vi "Client2.vi"() -> ()   [LabVIEW 2019]
panel:
  out "Connected":bool
  out "error out":errorcluster
  in  "UserName :":string
  in  "JOIN":bool
  in  "Message":string
  in  "SEND Button":bool
  in  "?":bool
  out "Chat Screen":string
  # "Welcome to Chat Application\nPlease type a username and click \"JOIN\" to join the chat room.\nYou can send your message  in \"Message Box\" with \"SEND MESSAGE\" button.\nAnd you can leave the chat room with \"QUIT\" button.\nIf you want to Join the chat room again, you should stop and run program again."
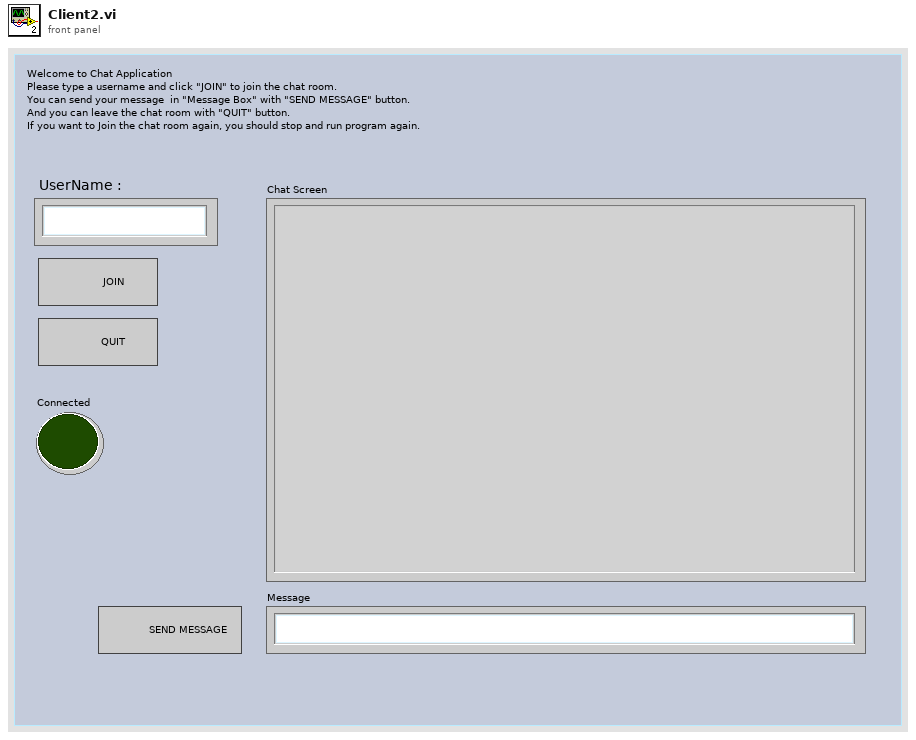
[diagram p1: front panel]
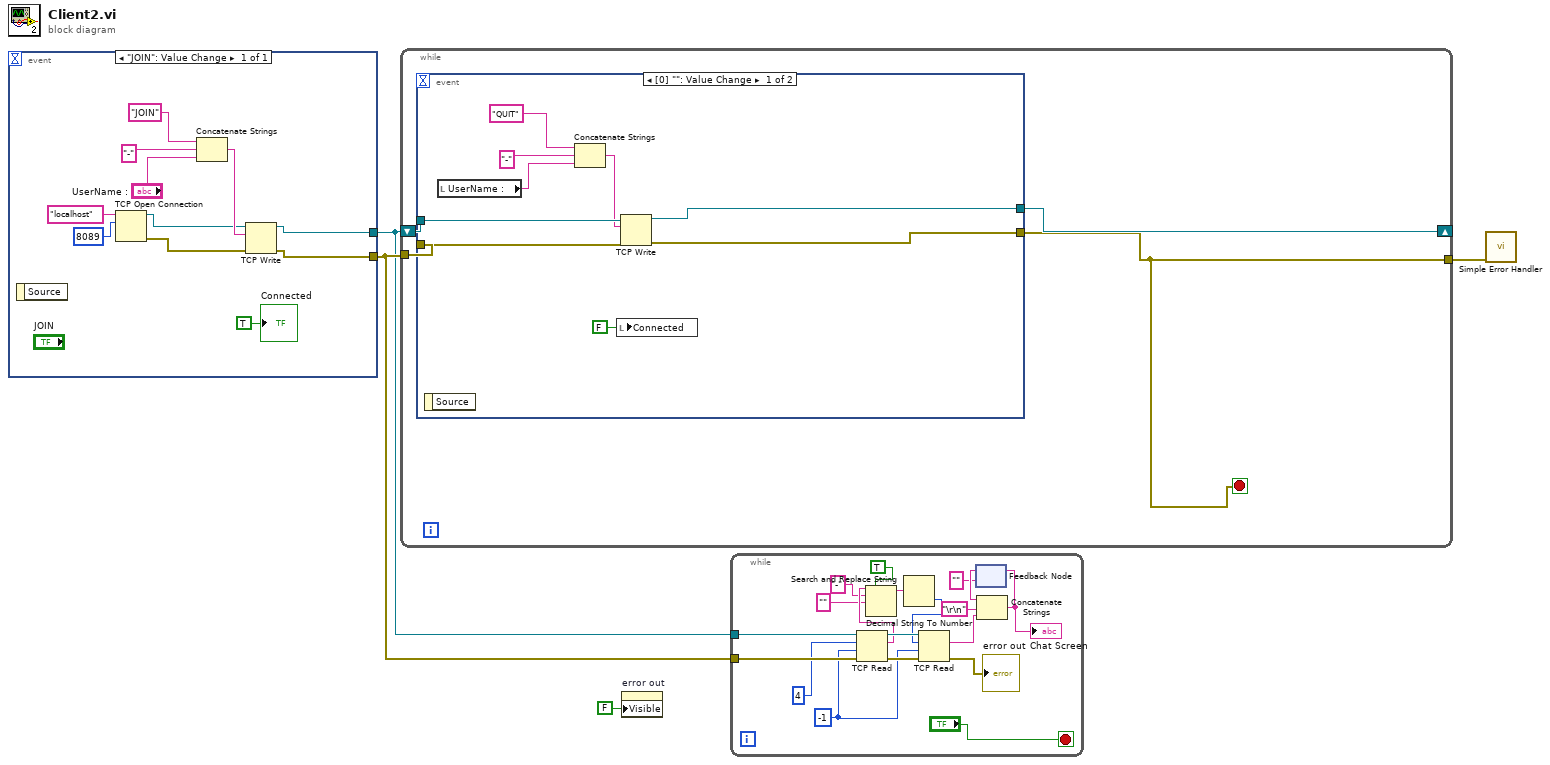
[diagram p0: block diagram]
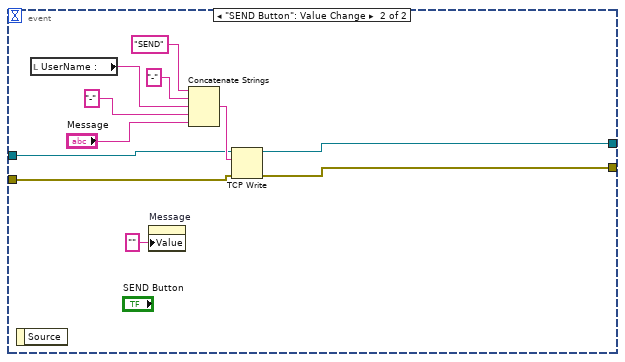
[diagram p2: hidden frame]
diagram:
  n1 = event shown="[0] \"JOIN\": Value Change" {
    selector: _ -> [_]
    dyn-events: _ -> [_]
    timeout: _ -> [_]
    tunnel: [w9] -> w4
    tunnel: [w10] -> w3
    event "JOIN": Value Change {
      n2 = event-data() -> ()  [unwired: 1 in, 1 out]
      n3 = TCP Open Connection(address="localhost", remote port or service name=u16 8089) -> (connection ID=w8:refnum<k5>, error out=w7:errorcluster)  [unwired: 3 in]
      n4 = Concatenate Strings("JOIN" ("data in"), "-" ("string"), "UserName :") -> (w13:string)
      n5 = TCP Write(connection ID=w8, data in=w13, error in (no error)=w7) -> (connection ID out=w10:refnum<k5>, error out=w9:errorcluster)  [unwired: 1 in, 1 out]
      "Connected" <- TRUE ("Connected")
    }
  }
  n6 = while {
    tunnel: w4 -> [w18]
    shift-right: [w17] -> _
    shift-left: w3 -> [w19]
    tunnel: [w16] -> w2
    stop <- w16 stop-if-true
    n7 = event shown="[0] \"\": Value Change" {
      selector: _ -> [_ _]
      dyn-events: _ -> [_ _]
      timeout: _ -> [_ _]
      tunnel: w18 -> [w27 w37]
      tunnel: w19 -> [w28 w38]
      tunnel: [w22 w30] -> w16
      tunnel: [w23 w31] -> w17
      event Value Change {
        n8 = event-data() -> ()  [unwired: 1 in, 1 out]
        n9 = local read "UserName :"() -> (w20:string)
        n10 = Concatenate Strings("QUIT" ("data in"), "-" ("string"), w20) -> (w24:string)
        n11 = local write "Connected"(FALSE ("Connected")) -> ()
        n12 = TCP Write(connection ID=w28, data in=w24, error in (no error)=w27) -> (connection ID out=w23:refnum<k5>, error out=w22:errorcluster)  [unwired: 1 in, 1 out]
      }
      event "SEND Button": Value Change {
        n13 = event-data() -> ()  [unwired: 1 in, 1 out]
        n14 = local read "UserName :"() -> (w33:string)
        n15 = property on="Message" class="Str"("Value"="" ("Message")) -> ()  [unwired: 2 in, 2 out]
        n16 = Concatenate Strings("SEND" ("string"), "-" ("string"), w33, "-" ("string"), "Message") -> (w39:string)
        n17 = TCP Write(connection ID=w38, data in=w39, error in (no error)=w37) -> (connection ID out=w31:refnum<k5>, error out=w30:errorcluster)  [unwired: 1 in, 1 out]
      }
    }
  }
  n18 = property on="error out" class="Clust (strict)"("Visible"=FALSE) -> ()  [unwired: 2 in, 2 out]
  n19 = while {
    tunnel: w4 -> [w58]
    tunnel: w3 -> [w57]
    stop <- "?" stop-if-true
    w47 = -1 ("timeout ms (25000)")
    n20 = TCP Read(connection ID=w57, bytes to read=4, error in (no error)=w58, 9:w47) -> (connection ID out=w56:refnum<k5>, data out=w54:string, error out=w52:errorcluster)  [unwired: 1 in]
    n21 = Search and Replace String(replace all?=TRUE ("replace all? (F)"), input string=w54, search string="-", replace string="" ("replace string (\"\")")) -> (result string=w55:string)  [unwired: 4 in, 3 out]
    n22 = Decimal String To Number(string=w55) -> (number=w53:i32)  [unwired: 2 in, 1 out]
    n23 = TCP Read(connection ID=w56, bytes to read=w53, error in (no error)=w52, 9:w47) -> (data out=w51:string, error out=→"error out":errorcluster)  [unwired: 1 in, 1 out]
    n24 = feedback #1("") -> (w44:string)
    n25 = Concatenate Strings(w44, "\r\n", w51) -> (w43:string)
    "Chat Screen" <- w43
    n26 = feedback-in #1(w43) -> ()
  }
  n27 = call <vilib>:"Simple Error Handler.vi"("error in (no error)"=w2) -> ()  [unwired: 4 in, 5 out]
